vi "(3) Built In Homing Function - All Axis.vi"() -> ()   [LabVIEW 2020]
uses:
  <instrlib>/Arcus Ethernet Driver 1.0.0/ArcusEthernetComm/classes/Controller/_Controller.lvclass
panel:
  in  "Home":bool
  out "Scanning Rig Disconnection":errorcluster={"status"=TRUE, "code"=0, "source"=""}
  in  "error in (no error)":errorcluster
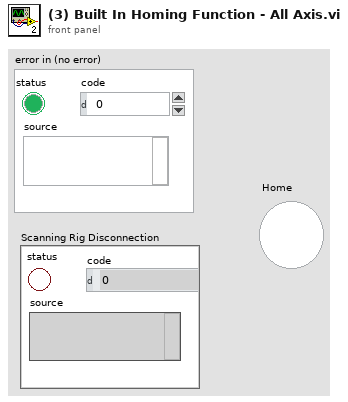
[diagram p1: front panel]
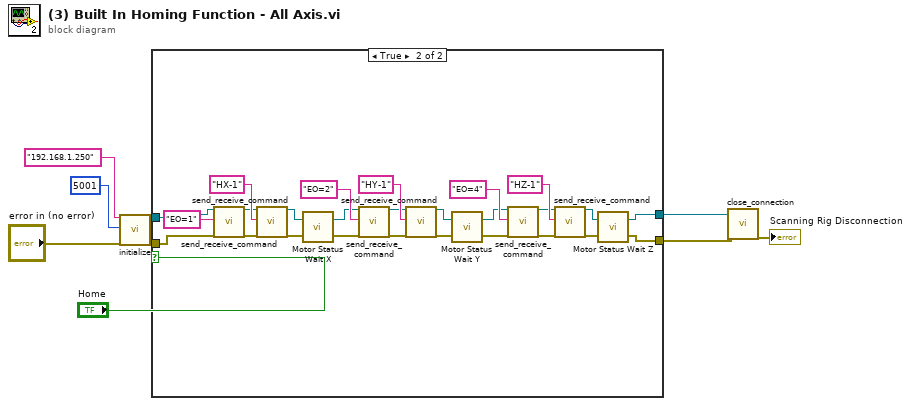
[diagram p0: block diagram]
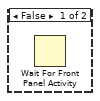
[diagram p2: hidden frame]
diagram:
  n1 = call <instrlib>:"initialize.vi"("ip_address (in)"="192.168.1.250", "dev_port(def=5001)"=u16 5001, "error in (no error)"="error in (no error)") -> ("reference (out)"=w5:refnum<class "_Controller.lvclass">, "error out"=w4:errorcluster)  [unwired: 15 in]
  n2 = case shown="True" "Home" {
    tunnel: w5 -> [_ w15]
    tunnel: w4 -> [_ w14]
    tunnel: [_ w10] -> w2
    tunnel: [_ w11] -> w1
    frame False {
      n3 = Wait For Front Panel Activity() -> ()  [unwired: 3 in, 1 out]
    }
    frame True {
      n4 = call <instrlib>:"send_receive_command.vi"("reference (in)"=w15, "ASCII Command (in)"="EO=1", "error in (no error)"=w14) -> ("reference (out)"=w23:refnum<class "_Controller.lvclass">, "error out"=w22:errorcluster)  [unwired: 12 in, 3 out]
      n5 = call <instrlib>:"send_receive_command.vi"("reference (in)"=w23, "ASCII Command (in)"="HX-1", "error in (no error)"=w22) -> ("reference (out)"=w32:refnum<class "_Controller.lvclass">, "error out"=w31:errorcluster)  [unwired: 12 in, 3 out]
      n6 = call "Motor Status Wait X.vi"("error in"=w31, "reference (in)"=w32) -> ("error out"=w21:errorcluster, "reference (out)"=w20:refnum<class "_Controller.lvclass">)
      n7 = call <instrlib>:"send_receive_command.vi"("reference (in)"=w20, "ASCII Command (in)"="EO=2", "error in (no error)"=w21) -> ("reference (out)"=w28:refnum<class "_Controller.lvclass">, "error out"=w27:errorcluster)  [unwired: 12 in, 3 out]
      n8 = call <instrlib>:"send_receive_command.vi"("reference (in)"=w28, "ASCII Command (in)"="HY-1", "error in (no error)"=w27) -> ("reference (out)"=w19:refnum<class "_Controller.lvclass">, "error out"=w18:errorcluster)  [unwired: 12 in, 3 out]
      n9 = call "Motor Status Wait Y.vi"("error in"=w18, "reference (in)"=w19) -> ("error out 2"=w17:errorcluster, "reference (out) 2"=w16:refnum<class "_Controller.lvclass">)
      n10 = call <instrlib>:"send_receive_command.vi"("reference (in)"=w16, "ASCII Command (in)"="EO=4", "error in (no error)"=w17) -> ("reference (out)"=w25:refnum<class "_Controller.lvclass">, "error out"=w24:errorcluster)  [unwired: 12 in, 3 out]
      n11 = call <instrlib>:"send_receive_command.vi"("reference (in)"=w25, "ASCII Command (in)"="HZ-1", "error in (no error)"=w24) -> ("reference (out)"=w13:refnum<class "_Controller.lvclass">, "error out"=w12:errorcluster)  [unwired: 12 in, 3 out]
      n12 = call "Motor Status Wait Z.vi"("error in"=w12, "reference (in)"=w13) -> ("error out 2"=w10:errorcluster, "reference (out) 2"=w11:refnum<class "_Controller.lvclass">)
    }
  }
  n13 = call <instrlib>:"close_connection.vi"("reference (in)"=w1, "error in (no error)"=w2) -> ("error out"=→"Scanning Rig Disconnection":errorcluster)  [unwired: 16 in, 1 out]
